vi "Find Resonances.vi"(8 "Error In":errorcluster) -> (0 "Error Out":errorcluster)   [LabVIEW 2016]
uses:
  Measure_extentions/Post-Processors/Line Detector/Line Detector Configuration.ctl
  Smooth Background CDBL.vi
  <vilib>/Analysis/NI_AALPro.lvlib
  <vilib>/Analysis/NI_AAL_SigProc.lvlib
  <vilib>/Analysis/NI_AALBase.lvlib
panel:
  out "XY Graph 6":cluster{dbl[], dbl[]}[](graph)
  in  "User configuration":T1={"Peak width"=30.0} {"Peak width" format="%#_6pHz"}
  in  "Signal channel":string="Signal"
  in  "Frequency channel":string="Frequency"
  in  "group name in":string="p"
  in  "HP F":dbl=0.1 format="%#_6p"
  in  "LP  F":dbl=0.001 format="%#_6p"
  in  "Fit?":bool
  in  "Complex":bool
  in  "Deviations":dbl=1.0
  out "variance":dbl format="%.2p"
  out "standard deviation":dbl format="%.2p"
  out "Peak F":dbl format="%#_6pHz"
  in  "Points around peak":i32=100
  in  "Peak number":i32
  out "XY Graph 5":cluster{"Array":dbl[], "Array":dbl[]}[](graph)
  out "width":i32=100 min=3
  out "XY Graph 4":cluster{"Y":dbl[], dbl[]}(graph)
  out "XY Graph 3":cluster{"Y":dbl[], "Y":dbl[]}[](graph)
  out "XY Graph 2":cluster{"Y":dbl[], dbl[]}[](graph)
  out "XY Graph":cluster{"Y":dbl[], "Unwrapped Phase":dbl[]}[](graph)
  in  "File Path Control":path=path "C:/Data/Spectra for Fedor/Ok spectra/300.00000K_175_555_2.10000V_0.00000T_May20-2015__09-37-18_001_052015.tdms"
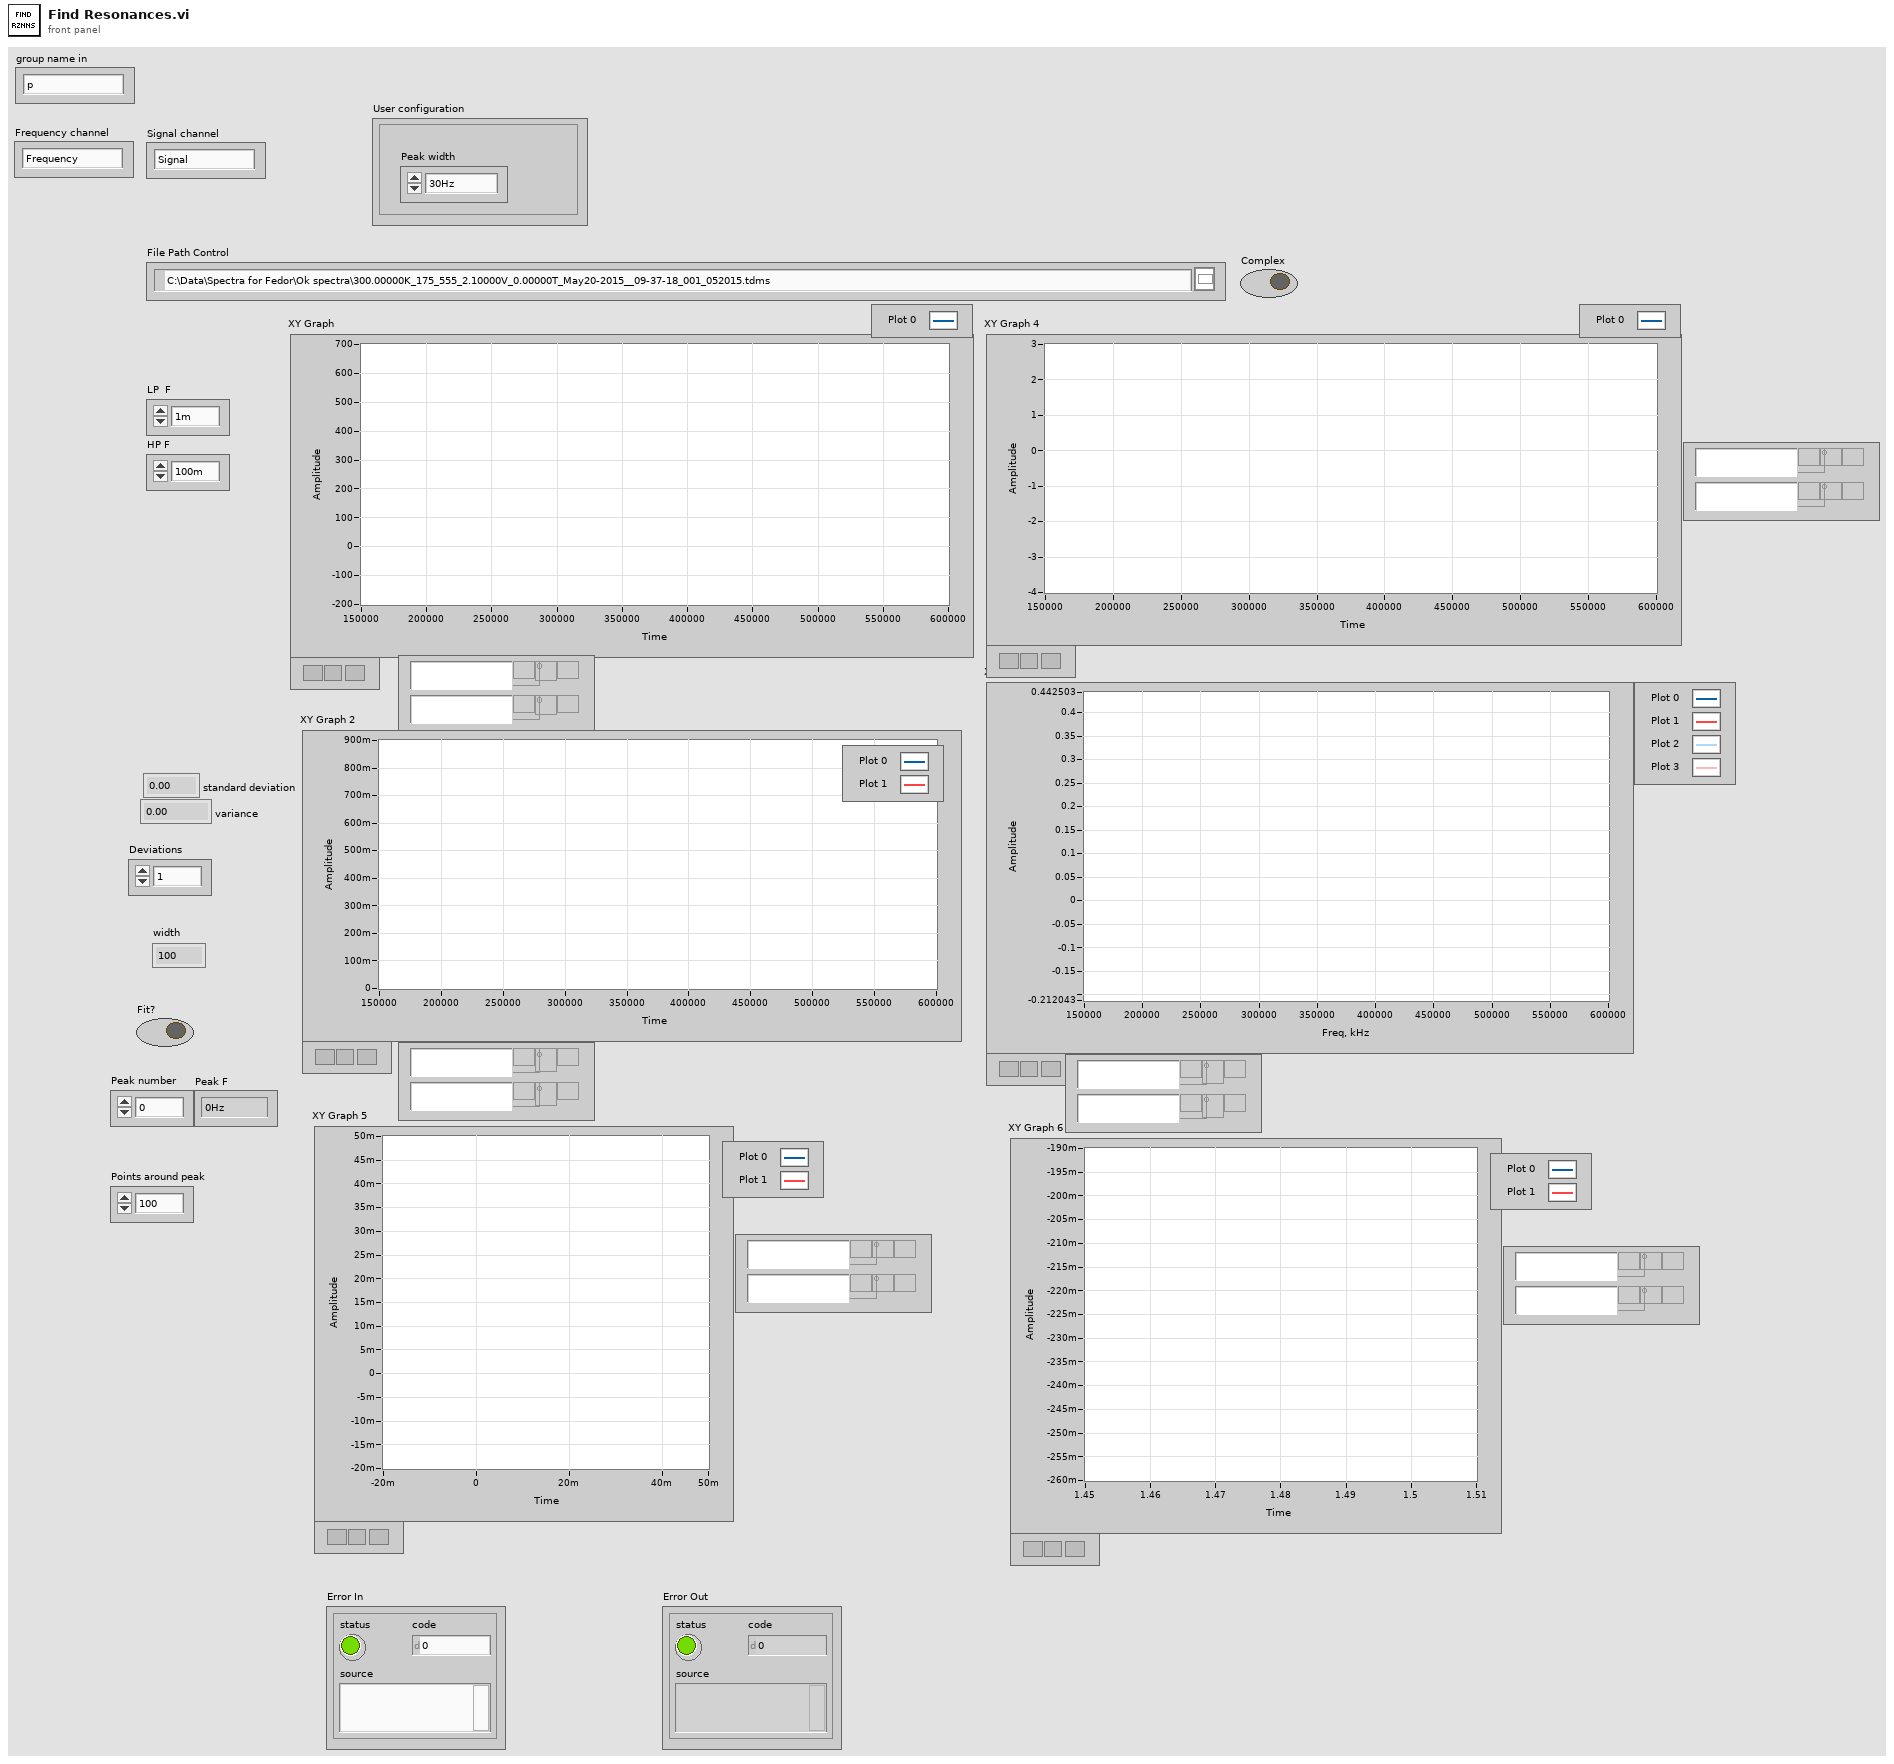
[diagram p1: front panel]
types:
  T1 = typedef "Line Detector Configuration.ctl" = cluster{"Peak width":dbl}
  T2 = enum16{"open", "open or create", "create or replace", "create", "open (read-only)"}
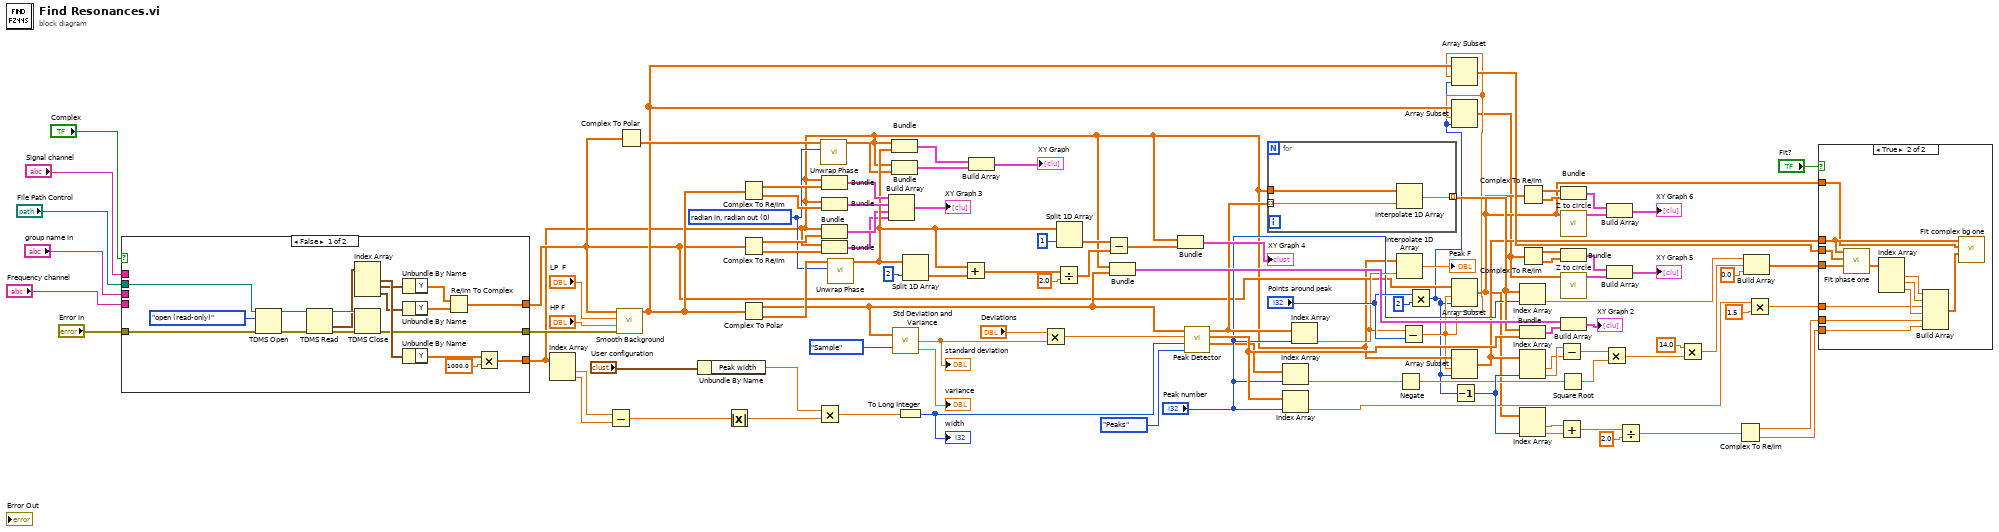
[diagram p0: block diagram]
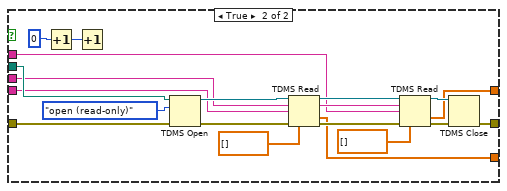
[diagram p3: hidden frame]
diagram:
  w67 = 0 items=["radian in, radian out", "radian in, degree out", "degree in, degree out", "degree in, radian out"] ("phase unit")
  n1 = case shown="False" "Complex" {
    tunnel: "File Path Control" -> [w123 w143]
    tunnel: [w107 w127] -> w24
    tunnel: "group name in" -> [_ w132]
    tunnel: "Frequency channel" -> [_ w131]
    tunnel: [w110 w128] -> w28
    tunnel: "Signal channel" -> [_ w126]
    tunnel: "Error In" -> [w109 w125]
    tunnel: [w108 w124] -> w25
    frame False {
      n2 = TDMS Open(8:w109, 10:T2."open (read-only)" ("operation (0:open)"), 11:w123) -> (0:w120:errorcluster, 3:w121:refnum<k34>)  [unwired: 4 in]
      n3 = TDMS Read(0:w121, 11:w120) -> (4:w119:refnum<k34>, 10:w117:waveform(dbl)[], 15:w118:errorcluster)  [unwired: 6 in, 3 out]
      n4 = Index Array(array=w117) -> (element #1=w116:waveform(dbl), element #2=w114:waveform(dbl), element #3=w115:waveform(dbl))  [unwired: 3 in]
      n5 = TDMS Close(8:w118, 11:w119) -> (0:w108:errorcluster)  [unwired: 1 out]
      n6 = Unbundle By Name(w114) -> ("Y"=w112:dbl[])
      n7 = Unbundle By Name(w115) -> ("Y"=w111:dbl[])
      n8 = Unbundle By Name(w116) -> ("Y"=w113:dbl[])
      n9 = Re/Im To Complex(1:w111, 2:w112) -> (0:w110:cdb[])
      n10 = Multiply(x=w113, y=1000.0) -> (x*y=w107:dbl[])
    }
    frame True {
      n11 = Increment(x=0 ("index")) -> (x+1=w137:i32)
      n12 = Increment(x=w137) -> ()  [unwired: 1 out]
      n13 = TDMS Open(8:w125, 10:T2."open (read-only)" ("operation (0:open)"), 11:w143) -> (0:w140:errorcluster, 3:w141:refnum<k34>)  [unwired: 4 in]
      n14 = TDMS Read(0:w141, 5:w132, 7:w131, 11:w140, 12:dbl[] []) -> (4:w135:refnum<k34>, 6:w133:string, 10:w127:dbl[], 15:w139:errorcluster)  [unwired: 3 in, 2 out]
      n15 = TDMS Read(0:w135, 5:w133, 7:w126, 11:w139, 12:cdb[] []) -> (4:w134:refnum<k34>, 10:w128:cdb[], 15:w136:errorcluster)  [unwired: 3 in, 3 out]
      n16 = TDMS Close(8:w136, 11:w134) -> (0:w124:errorcluster)  [unwired: 1 out]
    }
  }
  n17 = Index Array(array=w24) -> (element #1=w23:dbl, element #2=w22:dbl)  [unwired: 2 in]
  n18 = Subtract(x=w23, y=w22) -> (x-y=w21:dbl)
  n19 = call-poly "Smooth Background.vi"("Error In"=w25, "HP F"="HP F", "LP  F"="LP  F", "Data"=w28) -> ("Data out"=w37:cdb[])  [unwired: 6 in, 1 out]
  n20 = Complex To Polar(r * e^(i*theta)=w28) -> (theta=w66:dbl[])  [unwired: 1 out]
  n21 = Unbundle By Name("User configuration") -> ("Peak width"=w19:dbl)
  n22 = Absolute Value(x=w21) -> (abs(x)=w18:dbl)
  n23 = Complex To Re/Im(x + iy=w37) -> (x=w89:dbl[], y=w88:dbl[])
  n24 = Complex To Re/Im(x + iy=w28) -> (x=w77:dbl[], y=w78:dbl[])
  n25 = Complex To Polar(r * e^(i*theta)=w37) -> (r=w74:dbl[], theta=w95:dbl[])
  n26 = Multiply(x=w19, y=w18) -> (x*y=w17:dbl)
  n27 = call <vilib>:"Unwrap Phase.vi"("phase unit"=w67, "Phase"=w66) -> ("Unwrapped Phase"=w65:dbl[])  [unwired: 8 in, 1 out]
  n28 = Bundle(w24, w89) -> (w103:cluster{dbl[], dbl[]})  [unwired: 1 in]
  n29 = Bundle(w24, w88) -> (w102:cluster{dbl[], dbl[]})  [unwired: 1 in]
  n30 = Bundle(w24, w77) -> (w76:cluster{dbl[], dbl[]})  [unwired: 1 in]
  n31 = Bundle(w24, w78) -> (w75:cluster{dbl[], dbl[]})  [unwired: 1 in]
  n32 = call <vilib>:"Unwrap Phase.vi"("phase unit"=w67, "Phase"=w95) -> ("Unwrapped Phase"=w90:dbl[])  [unwired: 8 in, 1 out]
  n33 = Build Array(w103, w102, w76, w75) -> (→"XY Graph 3":cluster{dbl[], dbl[]}[])
  n34 = Bundle(w24, "Unwrapped Phase"=w90) -> (w104:cluster{dbl[], "Unwrapped Phase":dbl[]})  [unwired: 1 in]
  n35 = Bundle(w24, "Unwrapped Phase"=w65) -> (w63:cluster{dbl[], "Unwrapped Phase":dbl[]})  [unwired: 1 in]
  n36 = call <vilib>:"Std Deviation and Variance.vi"("X"=w74, "Weighting (Sample)"=enum16{"Sample", "Population"}."Sample") -> ("standard deviation"=w69:dbl, "variance"=→"variance":dbl)  [unwired: 1 out]
  "standard deviation" <- w69
  n37 = To Long Integer(number=w17) -> (32bit integer=w16:i32)
  "width" <- w16
  n38 = Split 1D Array(array=w90, index=2) -> (second subarray=w98:dbl[])  [unwired: 1 out]
  n39 = Add(x=w90, y=w98) -> (x+y=w97:dbl[])
  n40 = Build Array(w104, w63) -> (→"XY Graph":cluster{dbl[], "Unwrapped Phase":dbl[]}[])
  n41 = Multiply(x="Deviations", y=w69) -> (x*y=w70:dbl)
  n42 = Divide(x=w97, y=2.0) -> (x/y=w94:dbl[])
  n43 = Split 1D Array(array=w90, index=1) -> (second subarray=w91:dbl[])  [unwired: 1 out]
  n44 = Subtract(x=w91, y=w94) -> (x-y=w93:dbl[])
  n45 = Bundle(w24, w74) -> (w87:cluster{dbl[], dbl[]})  [unwired: 1 in]
  n46 = Bundle(w24, w93) -> (→"XY Graph 4":cluster{dbl[], dbl[]})  [unwired: 1 in]
  n47 = call <vilib>:"Peak Detector.vi"("peaks/valleys"=enum32{"Peaks", "Valleys"}."Peaks", "width"=w16, "threshold"=w70, "X"=w74) -> ("2nd Derivatives"=w53:dbl[], "Amplitudes"=w60:dbl[], "Locations"=w55:dbl[])  [unwired: 3 in, 2 out]
  n48 = for {
    tunnel: w24 -> [w146]
    tunnel: w55 -> [w145] mode=indexing
    tunnel: [w144] -> w59 mode=indexing
    n49 = Interpolate 1D Array(1:w145, 2:w146) -> (0:w144:dbl)
  }
  n50 = Index Array(array=w53, index="Peak number") -> (element=w52:dbl)
  n51 = Index Array(array=w60, index="Peak number") -> (element=w32:dbl)
  n52 = Index Array(array=w55, index="Peak number") -> (element=w61:dbl)
  n53 = Interpolate 1D Array(1:w61, 2:w24) -> (0:→"Peak F":dbl)
  n54 = Negate(x=w52) -> (-x=w49:dbl)
  n55 = Subtract(x=w61, y="Points around peak") -> (x-y=w13:dbl)
  n56 = Multiply(x="Points around peak", y=2) -> (x*y=w12:i32)
  n57 = Array Subset(array=w37, index=w13, length=w12) -> (w38:cdb[])
  n58 = Array Subset(array=w37, index=w13, length=w12) -> (w4:cdb[])
  n59 = Array Subset(array=w28, index=w13, length=w12) -> (w6:cdb[])
  n60 = Array Subset(array=w24, index=w13, length=w12) -> (w11:dbl[])
  n61 = Decrement(x=w12) -> (x-1=w58:i32)
  n62 = Index Array(array=w59, index="Peak number") -> (element=w45:dbl)
  n63 = Bundle(w59, "Amplitudes"=w60) -> (w84:cluster{dbl[], "Amplitudes":dbl[]})  [unwired: 1 in]
  n64 = Index Array(array=w11, index #2=w58) -> (element #1=w56:dbl, element #2=w57:dbl)  [unwired: 1 in]
  n65 = Index Array(array=w6, index #2=w58) -> (element #1=w48:cdb, element #2=w47:cdb)  [unwired: 1 in]
  n66 = Complex To Re/Im(x + iy=w6) -> (x=w9:dbl[], y=w8:dbl[])
  n67 = Complex To Re/Im(x + iy=w4) -> (x=w81:dbl[], y=w80:dbl[])
  n68 = Subtract(x=w57, y=w56) -> (x-y=w50:dbl)
  n69 = Add(x=w48, y=w47) -> (x+y=w46:cdb)
  n70 = Square Root(x=w49) -> (sqrt(x)=w51:dbl)
  n71 = Bundle(w9, w8) -> (w10:cluster{dbl[], dbl[]})  [unwired: 1 in]
  n72 = call "Z to circle.vi"("Z"=w6) -> ("plot"=w5:cluster{"Array":dbl[], "Array":dbl[]})  [unwired: 6 in, 4 out]
  n73 = Bundle(w81, w80) -> (w3:cluster{dbl[], dbl[]})  [unwired: 1 in]
  n74 = call "Z to circle.vi"("Z"=w4) -> ("plot"=w2:cluster{"Array":dbl[], "Array":dbl[]})  [unwired: 6 in, 4 out]
  n75 = Build Array(w87, w84) -> (→"XY Graph 2":cluster{dbl[], "Amplitudes":dbl[]}[])
  n76 = Multiply(x=w50, y=w51) -> (x*y=w44:dbl)
  n77 = Build Array(w10, w5) -> (→"XY Graph 6":cluster{"Array":dbl[], "Array":dbl[]}[])
  n78 = Build Array(w3, w2) -> (→"XY Graph 5":cluster{"Array":dbl[], "Array":dbl[]}[])
  n79 = Divide(x=w46, y=2.0) -> (x/y=w41:cdb)
  n80 = Multiply(x=14.0, y=w44) -> (x*y=w15:dbl)
  n81 = Complex To Re/Im(x + iy=w41) -> (x=w40:dbl, y=w39:dbl)
  n82 = Build Array(w45, w15, 0.0 ("element")) -> (w42:dbl[])
  n83 = Multiply(x=w32, y=1.5) -> (x*y=w31:dbl)
  n84 = case shown="True" "Fit?" {
    tunnel: w6 -> [_ w157]
    tunnel: w11 -> [_ w158]
    tunnel: w42 -> [_ w156]
    tunnel: w31 -> [_ w148]
    tunnel: w40 -> [_ w151]
    tunnel: w39 -> [_ w150]
    tunnel: w38 -> [_ w147]
    frame False {
    }
    frame True {
      n85 = call "Fit phase one.vi"("Initial parameters"=w156, "Z"=w147, "X"=w158) -> ("best fit parameters"=w155:dbl[])  [unwired: 8 in]
      n86 = Index Array(array=w155) -> (element #1=w154:dbl, element #2=w153:dbl, element #3=w152:dbl)  [unwired: 3 in]
      n87 = Build Array(w154, w153, w148, w152, w151, w150) -> (w149:dbl[])
      n88 = call "Fit complex bg one.vi"("Initial parameters"=w149, "Z"=w157, "X"=w158) -> ()  [unwired: 9 in]
    }
  }
